vi "Autonomous Independent.vi"() -> ()   [LabVIEW 2014]
doc: "This VI is called when autonomous begins, and will automatically be terminated when autonomous ends. You can carry out timed or sensor driven robot movement independently without needing to return to the caller."
uses:
  <vilib>/Rock Robotics/WPI/Joystick/WPI_JoystickGetSetRefNum.vi
panel:
  out "Stage 3":dbl
  out "Stage 8":dbl
  out "Stage 7":dbl
  out "Stage 6":dbl
  out "Stage 5":dbl
  out "Stage 4":dbl
  out "Stage 2":dbl
  out "Stage":dbl
  out "Right Distance 4":dbl
  out "Left Distance 4":dbl
  out "Elev Height 6":dbl
  out "Left Distance 6":dbl
  out "Right Distance 2":dbl
  out "Left Distance 2":dbl
  out "Right Distance 8":dbl
  out "Left Distance 8":dbl
  out "Right Distance 5":dbl
  out "Left Distance 5":dbl
  out "Right Distance 2":dbl
  out "Left Distance 2":dbl
  out "Right Distance":dbl
  out "Left Distance":dbl
  in  "Arm Control 3":bool
  in  "Right Side Speed 3":dbl
  in  "Left Side Speed 3":dbl
  in  "Elevator Height 4":dbl
  # "Be sure to right-click and choose Data Operations>>Make Current Value default if you want to save the array values with the VI"
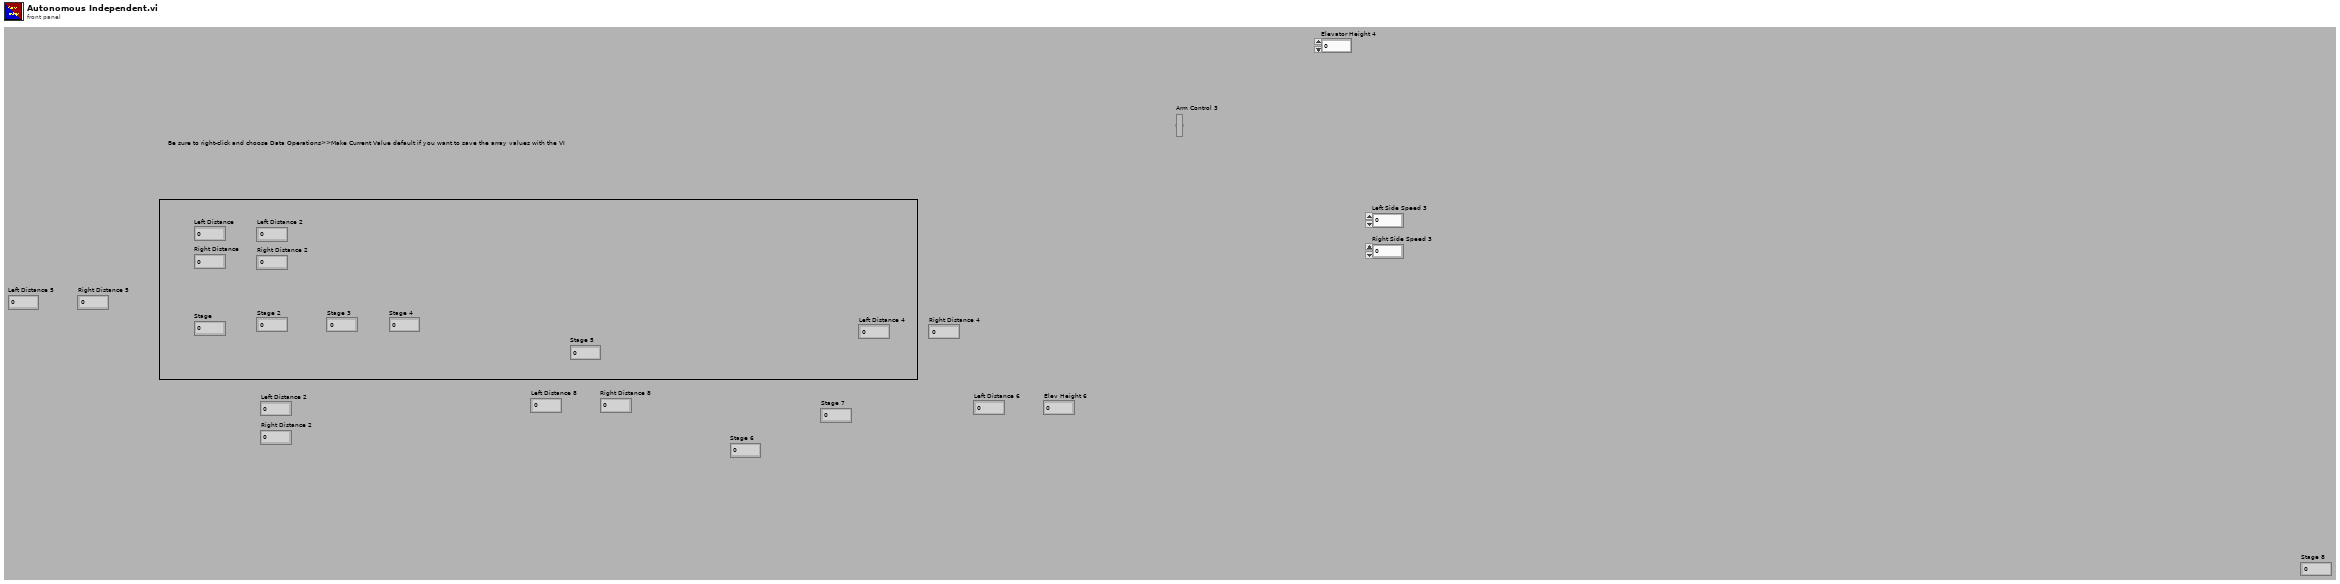
[diagram p1: front panel]
types:
  T1 = cluster{"Encoder Alarm Status":string, "Encoder Distance":dbl, "Encoder Direction":string, "Encoder Rate (distance/sec)":dbl}
  T2 = typedef "WPI_JoystickDevRef.ctl" = cluster{"Device":T3}
  T3 = typedef "WPI_JoystickDeviceEnum.ctl" = enum16{"USB 0", "USB 1", "USB 2", "USB 3", "USB 4", "USB 5"}
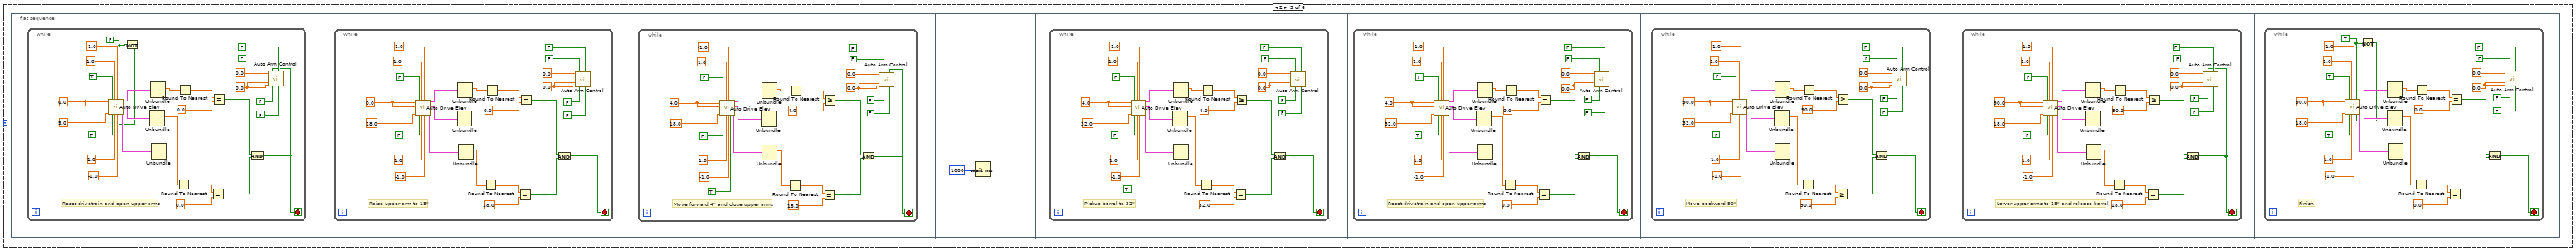
[diagram p3: hidden frame]
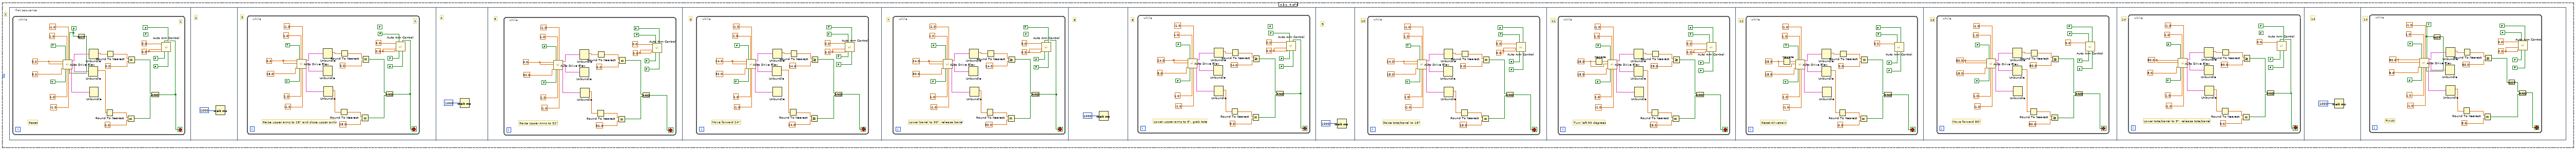
[diagram p4: hidden frame]
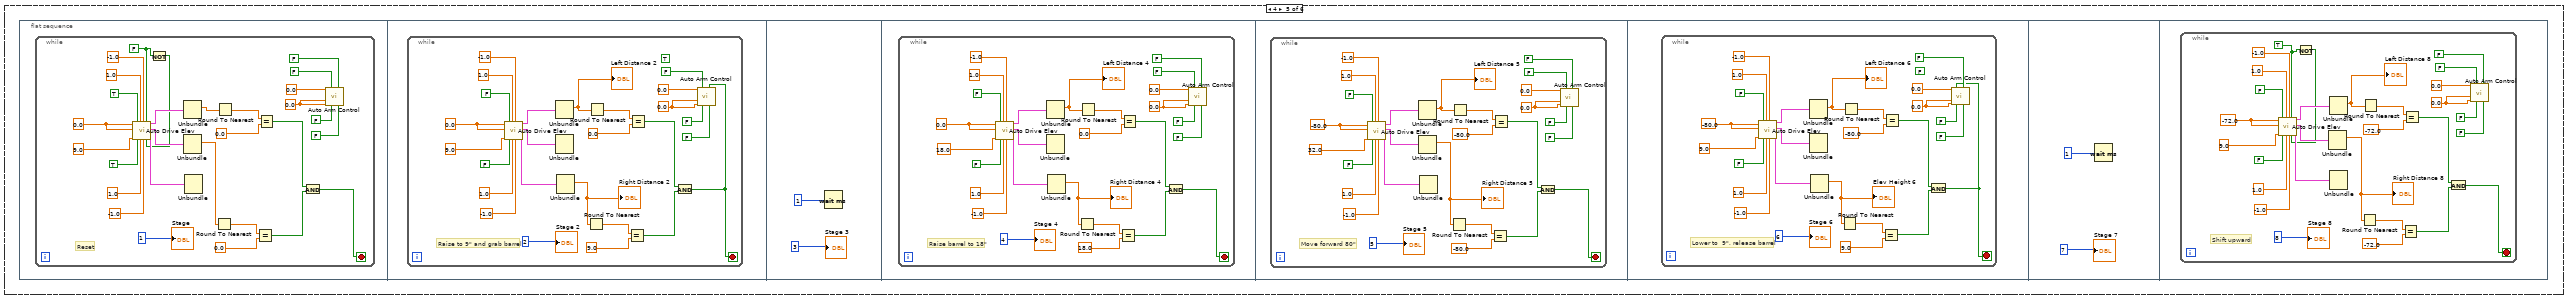
[diagram p5: hidden frame]
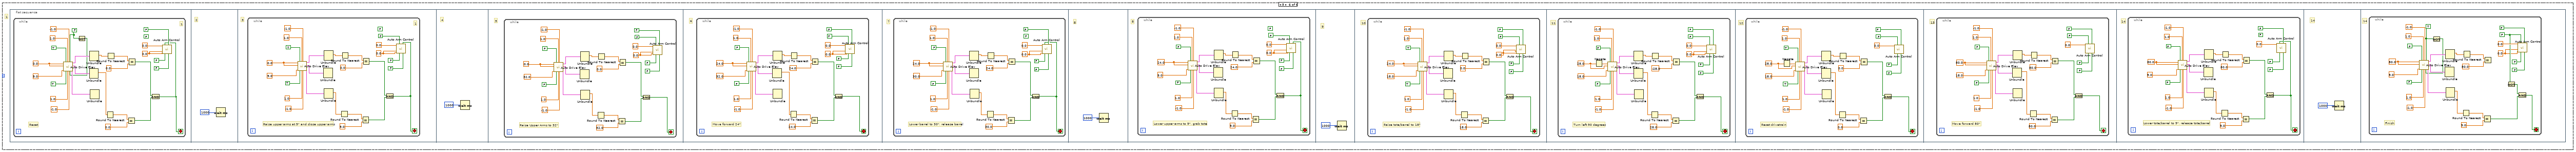
[diagram p6: hidden frame]
diagram:
  (unwired) "This function is run in parallel when the autonomous period begins. It will be terminated automatically when the period ends.\n\nNote that all Driver Station inputs are automatically latched and will not change once auto begins."
  # "Auto Modes\n\n0: Do Nothing\n1: Robot to AutoZone\n2: Barrel to AutoZone\n3: Barrel/Tote to AutoZone\n4: Barrel to AutoZone 2\n5: Discovery World"
  # "Every 20ms, report that we are running autonomous\ncode. Loop will abort the same time as the VI."
  # "This gives you the joystick value\nthat is often the throttle"
  # "This tells you the driver position\nand alliance color"
  n1 = case shown="1" 1 {
    frame 0, Default {
    }
    frame 1 {
      n2 = flat-sequence {
        frame #0 {
          n3 = while {
            stop <- w7 stop-if-true
            w11 = FALSE
            w14 = 0.0
            (unwired) FALSE
            w26 = 0.0
            # "Reset"
            n4 = Not(x=w11) -> (.not. x?=w10:bool)
            n5 = call "Auto Drive Elev.vi"("Left Side Speed"=w26, "Right Side Speed"=w26, "Elevator Height"=9.0, "Left Side Reset"=TRUE, "Right Side Reset"=TRUE, "Left Upper Limit"=1.0, "Right Upper Limit"=1.0, "Left Lower Limit"=-1.0, "Right Lower Limit"=-1.0, "Up Shift"=w11, "Down Shift"=w10) -> ("Encoder Status"=w24:T1, "Encoder Status 2"=w23:T1, "Encoder Status 3"=w22:T1)  [unwired: 6 in]
            n6 = Unbundle(w23) -> ("Encoder Distance"=w8:dbl)  [unwired: 3 out]
            "Right Distance" <- w8
            n7 = Unbundle(w24) -> ("Encoder Distance"=w9:dbl)  [unwired: 3 out]
            "Left Distance" <- w9
            n8 = Unbundle(w22) -> ()  [unwired: 4 out]
            n9 = Round To Nearest(number=w8) -> (nearest integer value=w20:dbl)
            n10 = Round To Nearest(number=w9) -> (nearest integer value=w17:dbl)
            n11 = Equal?(x=w20, y=0.0) -> (x = y?=w19:bool)
            n12 = Equal?(x=w17, y=0.0) -> (x = y?=w16:bool)
            n13 = And(x=w16, y=w19) -> (x .and. y?=w7:bool)
            n14 = call "Auto Arm Control.vi"("Upper Arm Rollers"=0.0, "Upper Arms Open"=FALSE, "Upper Arms Close"=w7, "Lower Roller Left"=w14, "Lower Roller Right"=w14, "Lower Arm Extend"=FALSE, "Lower Arm Retract"=FALSE) -> ()  [unwired: 9 in]
          }
        }
        frame #1 {
          n15 = while {
            stop <- w45 stop-if-true
            w37 = 0.0
            w52 = 60.0
            # "Move forward 5'"
            n16 = call "Auto Drive Elev.vi"("Left Side Speed"=w52, "Right Side Speed"=w52, "Elevator Height"=9.0, "Left Side Reset"=FALSE, "Right Side Reset"=FALSE, "Left Upper Limit"=0.3, "Right Upper Limit"=0.3, "Left Lower Limit"=-0.3, "Right Lower Limit"=-0.3) -> ("Encoder Status"=w50:T1, "Encoder Status 2"=w49:T1, "Encoder Status 3"=w48:T1)  [unwired: 8 in]
            n17 = Unbundle(w49) -> ("Encoder Distance"=w34:dbl)  [unwired: 3 out]
            n18 = Unbundle(w50) -> ("Encoder Distance"=w33:dbl)  [unwired: 3 out]
            n19 = Unbundle(w48) -> ()  [unwired: 4 out]
            n20 = Round To Nearest(number=w34) -> (nearest integer value=w46:dbl)
            n21 = Round To Nearest(number=w33) -> (nearest integer value=w42:dbl)
            n22 = Greater Or Equal?(x=w46, y=60.0) -> (x >= y?=w44:bool)
            n23 = Greater Or Equal?(x=w42, y=60.0) -> (x >= y?=w41:bool)
            n24 = And(x=w41, y=w44) -> (x .and. y?=w45:bool)
            n25 = call "Auto Arm Control.vi"("Upper Arm Rollers"=0.0, "Upper Arms Open"=FALSE, "Upper Arms Close"=FALSE, "Lower Roller Left"=w37, "Lower Roller Right"=w37, "Lower Arm Extend"=FALSE, "Lower Arm Retract"=FALSE) -> ()  [unwired: 9 in]
          }
        }
        frame #2 {
          n26 = while {
            stop <- w73 stop-if-true
            w60 = TRUE
            w65 = 0.0
            w80 = 60.0
            # "Shift upward"
            n27 = Not(x=w60) -> (.not. x?=w59:bool)
            n28 = call "Auto Drive Elev.vi"("Left Side Speed"=w80, "Right Side Speed"=w80, "Elevator Height"=9.0, "Left Side Reset"=FALSE, "Right Side Reset"=FALSE, "Left Upper Limit"=0.0, "Right Upper Limit"=0.0, "Left Lower Limit"=0.0, "Right Lower Limit"=0.0, "Up Shift"=w60, "Down Shift"=w59) -> ("Encoder Status"=w78:T1, "Encoder Status 2"=w77:T1, "Encoder Status 3"=w76:T1)  [unwired: 6 in]
            n29 = Unbundle(w77) -> ("Encoder Distance"=w62:dbl)  [unwired: 3 out]
            "Right Distance 2" <- w62
            n30 = Unbundle(w78) -> ("Encoder Distance"=w61:dbl)  [unwired: 3 out]
            "Left Distance 2" <- w61
            n31 = Unbundle(w76) -> ()  [unwired: 4 out]
            n32 = Round To Nearest(number=w62) -> (nearest integer value=w74:dbl)
            n33 = Round To Nearest(number=w61) -> (nearest integer value=w70:dbl)
            n34 = Greater Or Equal?(x=w74, y=60.0) -> (x >= y?=w72:bool)
            n35 = Greater Or Equal?(x=w70, y=60.0) -> (x >= y?=w69:bool)
            n36 = And(x=w69, y=w72) -> (x .and. y?=w73:bool)
            n37 = call "Auto Arm Control.vi"("Upper Arm Rollers"=0.0, "Upper Arms Open"=FALSE, "Upper Arms Close"=FALSE, "Lower Roller Left"=w65, "Lower Roller Right"=w65, "Lower Arm Extend"=FALSE, "Lower Arm Retract"=FALSE) -> ()  [unwired: 9 in]
          }
        }
      }
    }
    frame 2 {
      n38 = flat-sequence {
        frame #0 {
          n39 = while {
            stop <- w92 stop-if-true
            w88 = FALSE
            w89 = 0.0
            (unwired) FALSE
            w107 = 0.0
            # "Reset drivetrain and open upper arms"
            n40 = Not(x=w88) -> (.not. x?=w87:bool)
            n41 = call "Auto Drive Elev.vi"("Left Side Speed"=w107, "Right Side Speed"=w107, "Elevator Height"=9.0, "Left Side Reset"=TRUE, "Right Side Reset"=TRUE, "Left Upper Limit"=1.0, "Right Upper Limit"=1.0, "Left Lower Limit"=-1.0, "Right Lower Limit"=-1.0, "Up Shift"=w88, "Down Shift"=w87) -> ("Encoder Status"=w105:T1, "Encoder Status 2"=w104:T1, "Encoder Status 3"=w103:T1)  [unwired: 6 in]
            n42 = Unbundle(w104) -> ("Encoder Distance"=w100:dbl)  [unwired: 3 out]
            n43 = Unbundle(w105) -> ("Encoder Distance"=w96:dbl)  [unwired: 3 out]
            n44 = Unbundle(w103) -> ()  [unwired: 4 out]
            n45 = Round To Nearest(number=w100) -> (nearest integer value=w101:dbl)
            n46 = Round To Nearest(number=w96) -> (nearest integer value=w97:dbl)
            n47 = Equal?(x=w101, y=0.0) -> (x = y?=w99:bool)
            n48 = Equal?(x=w97, y=0.0) -> (x = y?=w95:bool)
            n49 = And(x=w95, y=w99) -> (x .and. y?=w92:bool)
            n50 = call "Auto Arm Control.vi"("Upper Arm Rollers"=0.0, "Upper Arms Open"=w92, "Upper Arms Close"=FALSE, "Lower Roller Left"=w89, "Lower Roller Right"=w89, "Lower Arm Extend"=FALSE, "Lower Arm Retract"=FALSE) -> ()  [unwired: 9 in]
          }
        }
        frame #1 {
          n51 = while {
            stop <- w126 stop-if-true
            w114 = 0.0
            w133 = 0.0
            # "Raise upper arm to 18\""
            n52 = call "Auto Drive Elev.vi"("Left Side Speed"=w133, "Right Side Speed"=w133, "Elevator Height"=18.0, "Left Side Reset"=FALSE, "Right Side Reset"=FALSE, "Left Upper Limit"=1.0, "Right Upper Limit"=1.0, "Left Lower Limit"=-1.0, "Right Lower Limit"=-1.0) -> ("Encoder Status"=w131:T1, "Encoder Status 2"=w130:T1, "Encoder Status 3"=w129:T1)  [unwired: 8 in]
            n53 = Unbundle(w130) -> ()  [unwired: 4 out]
            n54 = Unbundle(w131) -> ("Encoder Distance"=w122:dbl)  [unwired: 3 out]
            n55 = Unbundle(w129) -> ("Encoder Distance"=w117:dbl)  [unwired: 3 out]
            n56 = Round To Nearest(number=w117) -> (nearest integer value=w127:dbl)
            n57 = Round To Nearest(number=w122) -> (nearest integer value=w123:dbl)
            n58 = Equal?(x=w127, y=18.0) -> (x = y?=w125:bool)
            n59 = Equal?(x=w123, y=0.0) -> (x = y?=w121:bool)
            n60 = And(x=w121, y=w125) -> (x .and. y?=w126:bool)
            n61 = call "Auto Arm Control.vi"("Upper Arm Rollers"=0.0, "Upper Arms Open"=FALSE, "Upper Arms Close"=FALSE, "Lower Roller Left"=w114, "Lower Roller Right"=w114, "Lower Arm Extend"=FALSE, "Lower Arm Retract"=FALSE) -> ()  [unwired: 9 in]
          }
        }
        frame #2 {
          n62 = while {
            stop <- w144 stop-if-true
            w143 = 0.0
            (unwired) FALSE
            w159 = 4.0
            # "Move forward 4\" and close upper arms"
            n63 = call "Auto Drive Elev.vi"("Left Side Speed"=w159, "Right Side Speed"=w159, "Elevator Height"=18.0, "Left Side Reset"=FALSE, "Right Side Reset"=FALSE, "Left Upper Limit"=1.0, "Right Upper Limit"=1.0, "Left Lower Limit"=-1.0, "Right Lower Limit"=-1.0, "Down Shift"=TRUE) -> ("Encoder Status"=w157:T1, "Encoder Status 2"=w156:T1, "Encoder Status 3"=w155:T1)  [unwired: 7 in]
            n64 = Unbundle(w156) -> ()  [unwired: 4 out]
            n65 = Unbundle(w157) -> ("Encoder Distance"=w149:dbl)  [unwired: 3 out]
            n66 = Unbundle(w155) -> ("Encoder Distance"=w145:dbl)  [unwired: 3 out]
            n67 = Round To Nearest(number=w145) -> (nearest integer value=w153:dbl)
            n68 = Round To Nearest(number=w149) -> (nearest integer value=w150:dbl)
            n69 = Equal?(x=w153, y=18.0) -> (x = y?=w152:bool)
            n70 = Greater Or Equal?(x=w150, y=4.0) -> (x >= y?=w148:bool)
            n71 = And(x=w148, y=w152) -> (x .and. y?=w144:bool)
            n72 = call "Auto Arm Control.vi"("Upper Arm Rollers"=0.0, "Upper Arms Open"=FALSE, "Upper Arms Close"=w144, "Lower Roller Left"=w143, "Lower Roller Right"=w143, "Lower Arm Extend"=FALSE, "Lower Arm Retract"=FALSE) -> ()  [unwired: 9 in]
          }
        }
        frame #3 {
          n73 = Wait (ms)(milliseconds to wait=1000) -> ()  [unwired: 1 out]
        }
        frame #4 {
          n74 = while {
            stop <- w173 stop-if-true
            w170 = 0.0
            w187 = 4.0
            # "Pickup barrel to 32\""
            n75 = call "Auto Drive Elev.vi"("Left Side Speed"=w187, "Right Side Speed"=w187, "Elevator Height"=32.0, "Left Side Reset"=FALSE, "Right Side Reset"=FALSE, "Left Upper Limit"=1.0, "Right Upper Limit"=1.0, "Left Lower Limit"=-1.0, "Right Lower Limit"=-1.0, "Down Shift"=TRUE) -> ("Encoder Status"=w185:T1, "Encoder Status 2"=w184:T1, "Encoder Status 3"=w183:T1)  [unwired: 7 in]
            n76 = Unbundle(w184) -> ("Encoder Distance"=w172:dbl)  [unwired: 3 out]
            n77 = Unbundle(w185) -> ("Encoder Distance"=w177:dbl)  [unwired: 3 out]
            n78 = Unbundle(w183) -> ()  [unwired: 4 out]
            n79 = Round To Nearest(number=w172) -> (nearest integer value=w181:dbl)
            n80 = Round To Nearest(number=w177) -> (nearest integer value=w178:dbl)
            n81 = Equal?(x=w181, y=32.0) -> (x = y?=w180:bool)
            n82 = Greater Or Equal?(x=w178, y=4.0) -> (x >= y?=w176:bool)
            n83 = And(x=w176, y=w180) -> (x .and. y?=w173:bool)
            n84 = call "Auto Arm Control.vi"("Upper Arm Rollers"=0.0, "Upper Arms Open"=FALSE, "Upper Arms Close"=FALSE, "Lower Roller Left"=w170, "Lower Roller Right"=w170, "Lower Arm Extend"=FALSE, "Lower Arm Retract"=FALSE) -> ()  [unwired: 9 in]
          }
        }
        frame #5 {
          n85 = while {
            stop <- w198 stop-if-true
            w194 = 0.0
            w213 = 4.0
            # "Reset drivetrain and open upper arms"
            n86 = call "Auto Drive Elev.vi"("Left Side Speed"=w213, "Right Side Speed"=w213, "Elevator Height"=32.0, "Left Side Reset"=TRUE, "Right Side Reset"=TRUE, "Left Upper Limit"=1.0, "Right Upper Limit"=1.0, "Left Lower Limit"=-1.0, "Right Lower Limit"=-1.0) -> ("Encoder Status"=w211:T1, "Encoder Status 2"=w210:T1, "Encoder Status 3"=w209:T1)  [unwired: 8 in]
            n87 = Unbundle(w210) -> ("Encoder Distance"=w206:dbl)  [unwired: 3 out]
            n88 = Unbundle(w211) -> ("Encoder Distance"=w202:dbl)  [unwired: 3 out]
            n89 = Unbundle(w209) -> ()  [unwired: 4 out]
            n90 = Round To Nearest(number=w206) -> (nearest integer value=w207:dbl)
            n91 = Round To Nearest(number=w202) -> (nearest integer value=w203:dbl)
            n92 = Equal?(x=w207, y=0.0) -> (x = y?=w205:bool)
            n93 = Equal?(x=w203, y=0.0) -> (x = y?=w201:bool)
            n94 = And(x=w201, y=w205) -> (x .and. y?=w198:bool)
            n95 = call "Auto Arm Control.vi"("Upper Arm Rollers"=0.0, "Upper Arms Open"=FALSE, "Upper Arms Close"=FALSE, "Lower Roller Left"=w194, "Lower Roller Right"=w194, "Lower Arm Extend"=FALSE, "Lower Arm Retract"=FALSE) -> ()  [unwired: 9 in]
          }
        }
        frame #6 {
          n96 = while {
            stop <- w225 stop-if-true
            w222 = 0.0
            w239 = 90.0
            # "Move backward 90\""
            n97 = call "Auto Drive Elev.vi"("Left Side Speed"=w239, "Right Side Speed"=w239, "Elevator Height"=32.0, "Left Side Reset"=FALSE, "Right Side Reset"=FALSE, "Left Upper Limit"=1.0, "Right Upper Limit"=1.0, "Left Lower Limit"=-1.0, "Right Lower Limit"=-1.0) -> ("Encoder Status"=w237:T1, "Encoder Status 2"=w236:T1, "Encoder Status 3"=w235:T1)  [unwired: 8 in]
            n98 = Unbundle(w236) -> ("Encoder Distance"=w223:dbl)  [unwired: 3 out]
            n99 = Unbundle(w237) -> ("Encoder Distance"=w229:dbl)  [unwired: 3 out]
            n100 = Unbundle(w235) -> ()  [unwired: 4 out]
            n101 = Round To Nearest(number=w223) -> (nearest integer value=w233:dbl)
            n102 = Round To Nearest(number=w229) -> (nearest integer value=w230:dbl)
            n103 = Greater Or Equal?(x=w233, y=90.0) -> (x >= y?=w232:bool)
            n104 = Greater Or Equal?(x=w230, y=90.0) -> (x >= y?=w228:bool)
            n105 = And(x=w228, y=w232) -> (x .and. y?=w225:bool)
            n106 = call "Auto Arm Control.vi"("Upper Arm Rollers"=0.0, "Upper Arms Open"=FALSE, "Upper Arms Close"=FALSE, "Lower Roller Left"=w222, "Lower Roller Right"=w222, "Lower Arm Extend"=FALSE, "Lower Arm Retract"=FALSE) -> ()  [unwired: 9 in]
          }
        }
        frame #7 {
          n107 = while {
            stop <- w249 stop-if-true
            w246 = 0.0
            (unwired) FALSE
            w264 = 90.0
            # "Lower upper arms to 18\" and release barrel"
            n108 = call "Auto Drive Elev.vi"("Left Side Speed"=w264, "Right Side Speed"=w264, "Elevator Height"=18.0, "Left Side Reset"=FALSE, "Right Side Reset"=FALSE, "Left Upper Limit"=1.0, "Right Upper Limit"=1.0, "Left Lower Limit"=-1.0, "Right Lower Limit"=-1.0) -> ("Encoder Status"=w262:T1, "Encoder Status 2"=w261:T1, "Encoder Status 3"=w260:T1)  [unwired: 8 in]
            n109 = Unbundle(w261) -> ()  [unwired: 4 out]
            n110 = Unbundle(w262) -> ("Encoder Distance"=w254:dbl)  [unwired: 3 out]
            n111 = Unbundle(w260) -> ("Encoder Distance"=w250:dbl)  [unwired: 3 out]
            n112 = Round To Nearest(number=w250) -> (nearest integer value=w258:dbl)
            n113 = Round To Nearest(number=w254) -> (nearest integer value=w255:dbl)
            n114 = Equal?(x=w258, y=18.0) -> (x = y?=w257:bool)
            n115 = Greater Or Equal?(x=w255, y=90.0) -> (x >= y?=w253:bool)
            n116 = And(x=w253, y=w257) -> (x .and. y?=w249:bool)
            n117 = call "Auto Arm Control.vi"("Upper Arm Rollers"=0.0, "Upper Arms Open"=w249, "Upper Arms Close"=FALSE, "Lower Roller Left"=w246, "Lower Roller Right"=w246, "Lower Arm Extend"=FALSE, "Lower Arm Retract"=FALSE) -> ()  [unwired: 9 in]
          }
        }
        frame #8 {
          n118 = while {
            stop <- w278 stop-if-true
            w271 = TRUE
            w273 = 0.0
            w292 = 90.0
            # "Finish"
            n119 = Not(x=w271) -> (.not. x?=w272:bool)
            n120 = call "Auto Drive Elev.vi"("Left Side Speed"=w292, "Right Side Speed"=w292, "Elevator Height"=18.0, "Left Side Reset"=TRUE, "Right Side Reset"=TRUE, "Left Upper Limit"=1.0, "Right Upper Limit"=1.0, "Left Lower Limit"=-1.0, "Right Lower Limit"=-1.0, "Up Shift"=w271, "Down Shift"=w272) -> ("Encoder Status"=w290:T1, "Encoder Status 2"=w289:T1, "Encoder Status 3"=w288:T1)  [unwired: 6 in]
            n121 = Unbundle(w289) -> ("Encoder Distance"=w277:dbl)  [unwired: 3 out]
            n122 = Unbundle(w290) -> ("Encoder Distance"=w282:dbl)  [unwired: 3 out]
            n123 = Unbundle(w288) -> ()  [unwired: 4 out]
            n124 = Round To Nearest(number=w277) -> (nearest integer value=w286:dbl)
            n125 = Round To Nearest(number=w282) -> (nearest integer value=w283:dbl)
            n126 = Equal?(x=w286, y=0.0) -> (x = y?=w285:bool)
            n127 = Equal?(x=w283, y=0.0) -> (x = y?=w281:bool)
            n128 = And(x=w281, y=w285) -> (x .and. y?=w278:bool)
            n129 = call "Auto Arm Control.vi"("Upper Arm Rollers"=0.0, "Upper Arms Open"=FALSE, "Upper Arms Close"=FALSE, "Lower Roller Left"=w273, "Lower Roller Right"=w273, "Lower Arm Extend"=FALSE, "Lower Arm Retract"=FALSE) -> ()  [unwired: 9 in]
          }
        }
      }
    }
    frame 3 {
      # "1"
      n130 = flat-sequence {
        frame #0 {
          # "1"
          n131 = while {
            stop <- w301 stop-if-true
            w299 = FALSE
            w303 = 0.0
            (unwired) FALSE
            w319 = 0.0
            # "Reset"
            n132 = Not(x=w299) -> (.not. x?=w300:bool)
            n133 = call "Auto Drive Elev.vi"("Left Side Speed"=w319, "Right Side Speed"=w319, "Elevator Height"=9.0, "Left Side Reset"=TRUE, "Right Side Reset"=TRUE, "Left Upper Limit"=1.0, "Right Upper Limit"=1.0, "Left Lower Limit"=-1.0, "Right Lower Limit"=-1.0, "Up Shift"=w299, "Down Shift"=w300) -> ("Encoder Status"=w317:T1, "Encoder Status 2"=w316:T1, "Encoder Status 3"=w315:T1)  [unwired: 6 in]
            n134 = Unbundle(w316) -> ("Encoder Distance"=w312:dbl)  [unwired: 3 out]
            n135 = Unbundle(w317) -> ("Encoder Distance"=w308:dbl)  [unwired: 3 out]
            n136 = Unbundle(w315) -> ()  [unwired: 4 out]
            n137 = Round To Nearest(number=w312) -> (nearest integer value=w313:dbl)
            n138 = Round To Nearest(number=w308) -> (nearest integer value=w309:dbl)
            n139 = Equal?(x=w313, y=0.0) -> (x = y?=w311:bool)
            n140 = Equal?(x=w309, y=0.0) -> (x = y?=w307:bool)
            n141 = And(x=w307, y=w311) -> (x .and. y?=w301:bool)
            n142 = call "Auto Arm Control.vi"("Upper Arm Rollers"=0.0, "Upper Arms Open"=w301, "Upper Arms Close"=FALSE, "Lower Roller Left"=w303, "Lower Roller Right"=w303, "Lower Arm Extend"=FALSE, "Lower Arm Retract"=FALSE) -> ()  [unwired: 9 in]
          }
        }
        frame #1 {
          # "2"
          n143 = Wait (ms)(milliseconds to wait=1000) -> ()  [unwired: 1 out]
        }
        frame #2 {
          # "3"
          # "1"
          n144 = while {
            stop <- w328 stop-if-true
            w329 = 0.0
            (unwired) FALSE
            w345 = 0.0
            # "Raise upper arms to 18\" and close upper arms"
            n145 = call "Auto Drive Elev.vi"("Left Side Speed"=w345, "Right Side Speed"=w345, "Elevator Height"=18.0, "Left Side Reset"=TRUE, "Right Side Reset"=TRUE, "Left Upper Limit"=1.0, "Right Upper Limit"=1.0, "Left Lower Limit"=-1.0, "Right Lower Limit"=-1.0) -> ("Encoder Status"=w343:T1, "Encoder Status 2"=w342:T1, "Encoder Status 3"=w341:T1)  [unwired: 8 in]
            n146 = Unbundle(w342) -> ()  [unwired: 4 out]
            n147 = Unbundle(w343) -> ("Encoder Distance"=w335:dbl)  [unwired: 3 out]
            n148 = Unbundle(w341) -> ("Encoder Distance"=w332:dbl)  [unwired: 3 out]
            n149 = Round To Nearest(number=w332) -> (nearest integer value=w339:dbl)
            n150 = Round To Nearest(number=w335) -> (nearest integer value=w336:dbl)
            n151 = Equal?(x=w339, y=18.0) -> (x = y?=w338:bool)
            n152 = Equal?(x=w336, y=0.0) -> (x = y?=w327:bool)
            n153 = And(x=w327, y=w338) -> (x .and. y?=w328:bool)
            n154 = call "Auto Arm Control.vi"("Upper Arm Rollers"=0.0, "Upper Arms Open"=FALSE, "Upper Arms Close"=w328, "Lower Roller Left"=w329, "Lower Roller Right"=w329, "Lower Arm Extend"=FALSE, "Lower Arm Retract"=FALSE) -> ()  [unwired: 9 in]
          }
        }
        frame #3 {
          # "4"
          n155 = Wait (ms)(milliseconds to wait=1000) -> ()  [unwired: 1 out]
        }
        frame #4 {
          # "5"
          n156 = while {
            stop <- w365 stop-if-true
            w354 = 0.0
            w372 = 0.0
            # "Raise Upper Arms to 32\""
            n157 = call "Auto Drive Elev.vi"("Left Side Speed"=w372, "Right Side Speed"=w372, "Elevator Height"=32.0, "Left Side Reset"=FALSE, "Right Side Reset"=FALSE, "Left Upper Limit"=1.0, "Right Upper Limit"=1.0, "Left Lower Limit"=-1.0, "Right Lower Limit"=-1.0) -> ("Encoder Status"=w370:T1, "Encoder Status 2"=w369:T1, "Encoder Status 3"=w368:T1)  [unwired: 8 in]
            n158 = Unbundle(w369) -> ()  [unwired: 4 out]
            n159 = Unbundle(w370) -> ("Encoder Distance"=w361:dbl)  [unwired: 3 out]
            n160 = Unbundle(w368) -> ("Encoder Distance"=w356:dbl)  [unwired: 3 out]
            n161 = Round To Nearest(number=w356) -> (nearest integer value=w366:dbl)
            n162 = Round To Nearest(number=w361) -> (nearest integer value=w362:dbl)
            n163 = Equal?(x=w366, y=32.0) -> (x = y?=w364:bool)
            n164 = Equal?(x=w362, y=0.0) -> (x = y?=w360:bool)
            n165 = And(x=w360, y=w364) -> (x .and. y?=w365:bool)
            n166 = call "Auto Arm Control.vi"("Upper Arm Rollers"=0.0, "Upper Arms Open"=FALSE, "Upper Arms Close"=FALSE, "Lower Roller Left"=w354, "Lower Roller Right"=w354, "Lower Arm Extend"=FALSE, "Lower Arm Retract"=FALSE) -> ()  [unwired: 9 in]
          }
        }
        frame #5 {
          # "6"
          n167 = while {
            stop <- w390 stop-if-true
            w379 = 0.0
            w398 = 24.0
            # "Move forward 24\""
            n168 = call "Auto Drive Elev.vi"("Left Side Speed"=w398, "Right Side Speed"=w398, "Elevator Height"=32.0, "Left Side Reset"=FALSE, "Right Side Reset"=FALSE, "Left Upper Limit"=1.0, "Right Upper Limit"=1.0, "Left Lower Limit"=-1.0, "Right Lower Limit"=-1.0) -> ("Encoder Status"=w396:T1, "Encoder Status 2"=w395:T1, "Encoder Status 3"=w394:T1)  [unwired: 8 in]
            n169 = Unbundle(w395) -> ("Encoder Distance"=w391:dbl)  [unwired: 3 out]
            n170 = Unbundle(w396) -> ("Encoder Distance"=w386:dbl)  [unwired: 3 out]
            n171 = Unbundle(w394) -> ()  [unwired: 4 out]
            n172 = Round To Nearest(number=w391) -> (nearest integer value=w392:dbl)
            n173 = Round To Nearest(number=w386) -> (nearest integer value=w387:dbl)
            n174 = Greater Or Equal?(x=w392, y=24.0) -> (x >= y?=w389:bool)
            n175 = Greater Or Equal?(x=w387, y=24.0) -> (x >= y?=w385:bool)
            n176 = And(x=w385, y=w389) -> (x .and. y?=w390:bool)
            n177 = call "Auto Arm Control.vi"("Upper Arm Rollers"=0.0, "Upper Arms Open"=FALSE, "Upper Arms Close"=FALSE, "Lower Roller Left"=w379, "Lower Roller Right"=w379, "Lower Arm Extend"=FALSE, "Lower Arm Retract"=FALSE) -> ()  [unwired: 9 in]
          }
        }
        frame #6 {
          # "7"
          n178 = while {
            stop <- w405 stop-if-true
            w406 = 0.0
            (unwired) FALSE
            w423 = 24.0
            # "Lower barrel to 30\", release barrel"
            n179 = call "Auto Drive Elev.vi"("Left Side Speed"=w423, "Right Side Speed"=w423, "Elevator Height"=30.0, "Left Side Reset"=FALSE, "Right Side Reset"=FALSE, "Left Upper Limit"=1.0, "Right Upper Limit"=1.0, "Left Lower Limit"=-1.0, "Right Lower Limit"=-1.0) -> ("Encoder Status"=w421:T1, "Encoder Status 2"=w420:T1, "Encoder Status 3"=w419:T1)  [unwired: 8 in]
            n180 = Unbundle(w420) -> ()  [unwired: 4 out]
            n181 = Unbundle(w421) -> ("Encoder Distance"=w413:dbl)  [unwired: 3 out]
            n182 = Unbundle(w419) -> ("Encoder Distance"=w409:dbl)  [unwired: 3 out]
            n183 = Round To Nearest(number=w409) -> (nearest integer value=w417:dbl)
            n184 = Round To Nearest(number=w413) -> (nearest integer value=w414:dbl)
            n185 = Equal?(x=w417, y=30.0) -> (x = y?=w416:bool)
            n186 = Greater Or Equal?(x=w414, y=24.0) -> (x >= y?=w412:bool)
            n187 = And(x=w412, y=w416) -> (x .and. y?=w405:bool)
            n188 = call "Auto Arm Control.vi"("Upper Arm Rollers"=0.0, "Upper Arms Open"=w405, "Upper Arms Close"=FALSE, "Lower Roller Left"=w406, "Lower Roller Right"=w406, "Lower Arm Extend"=FALSE, "Lower Arm Retract"=FALSE) -> ()  [unwired: 9 in]
          }
        }
        frame #7 {
          # "8"
          n189 = Wait (ms)(milliseconds to wait=1000) -> ()  [unwired: 1 out]
        }
        frame #8 {
          # "8"
          n190 = while {
            stop <- w431 stop-if-true
            w434 = 0.0
            (unwired) FALSE
            w449 = 24.0
            # "Lower upper arms to 9\", grab tote"
            n191 = call "Auto Drive Elev.vi"("Left Side Speed"=w449, "Right Side Speed"=w449, "Elevator Height"=9.0, "Left Side Reset"=FALSE, "Right Side Reset"=FALSE, "Left Upper Limit"=1.0, "Right Upper Limit"=1.0, "Left Lower Limit"=-1.0, "Right Lower Limit"=-1.0) -> ("Encoder Status"=w447:T1, "Encoder Status 2"=w446:T1, "Encoder Status 3"=w445:T1)  [unwired: 8 in]
            n192 = Unbundle(w446) -> ()  [unwired: 4 out]
            n193 = Unbundle(w447) -> ("Encoder Distance"=w439:dbl)  [unwired: 3 out]
            n194 = Unbundle(w445) -> ("Encoder Distance"=w435:dbl)  [unwired: 3 out]
            n195 = Round To Nearest(number=w435) -> (nearest integer value=w443:dbl)
            n196 = Round To Nearest(number=w439) -> (nearest integer value=w440:dbl)
            n197 = Equal?(x=w443, y=9.0) -> (x = y?=w442:bool)
            n198 = Greater Or Equal?(x=w440, y=24.0) -> (x >= y?=w438:bool)
            n199 = And(x=w438, y=w442) -> (x .and. y?=w431:bool)
            n200 = call "Auto Arm Control.vi"("Upper Arm Rollers"=0.0, "Upper Arms Open"=FALSE, "Upper Arms Close"=w431, "Lower Roller Left"=w434, "Lower Roller Right"=w434, "Lower Arm Extend"=FALSE, "Lower Arm Retract"=FALSE) -> ()  [unwired: 9 in]
          }
        }
        frame #9 {
          # "9"
          n201 = Wait (ms)(milliseconds to wait=1000) -> ()  [unwired: 1 out]
        }
        frame #10 {
          # "10"
          n202 = while {
            stop <- w469 stop-if-true
            w457 = 0.0
            w476 = 24.0
            # "Raise tote/barrel to 18\""
            n203 = call "Auto Drive Elev.vi"("Left Side Speed"=w476, "Right Side Speed"=w476, "Elevator Height"=18.0, "Left Side Reset"=TRUE, "Right Side Reset"=TRUE, "Left Upper Limit"=1.0, "Right Upper Limit"=1.0, "Left Lower Limit"=-1.0, "Right Lower Limit"=-1.0) -> ("Encoder Status"=w474:T1, "Encoder Status 2"=w473:T1, "Encoder Status 3"=w472:T1)  [unwired: 8 in]
            n204 = Unbundle(w473) -> ()  [unwired: 4 out]
            n205 = Unbundle(w474) -> ("Encoder Distance"=w465:dbl)  [unwired: 3 out]
            n206 = Unbundle(w472) -> ("Encoder Distance"=w460:dbl)  [unwired: 3 out]
            n207 = Round To Nearest(number=w460) -> (nearest integer value=w470:dbl)
            n208 = Round To Nearest(number=w465) -> (nearest integer value=w466:dbl)
            n209 = Equal?(x=w470, y=18.0) -> (x = y?=w468:bool)
            n210 = Equal?(x=w466, y=0.0) -> (x = y?=w461:bool)
            n211 = And(x=w461, y=w468) -> (x .and. y?=w469:bool)
            n212 = call "Auto Arm Control.vi"("Upper Arm Rollers"=0.0, "Upper Arms Open"=FALSE, "Upper Arms Close"=FALSE, "Lower Roller Left"=w457, "Lower Roller Right"=w457, "Lower Arm Extend"=FALSE, "Lower Arm Retract"=FALSE) -> ()  [unwired: 9 in]
          }
        }
        frame #11 {
          # "11"
          n213 = while {
            stop <- w497 stop-if-true
            w483 = 0.0
            w486 = 28.0
            # "Turn left 90 degrees"
            n214 = Negate(x=w486) -> (-x=w487:dbl)
            n215 = call "Auto Drive Elev.vi"("Left Side Speed"=w487, "Right Side Speed"=w486, "Elevator Height"=18.0, "Left Side Reset"=FALSE, "Right Side Reset"=FALSE, "Left Upper Limit"=1.0, "Right Upper Limit"=1.0, "Left Lower Limit"=-1.0, "Right Lower Limit"=-1.0) -> ("Encoder Status"=w502:T1, "Encoder Status 2"=w501:T1, "Encoder Status 3"=w500:T1)  [unwired: 8 in]
            n216 = Unbundle(w501) -> ("Encoder Distance"=w488:dbl)  [unwired: 3 out]
            n217 = Unbundle(w502) -> ("Encoder Distance"=w493:dbl)  [unwired: 3 out]
            n218 = Unbundle(w500) -> ()  [unwired: 4 out]
            n219 = Round To Nearest(number=w488) -> (nearest integer value=w498:dbl)
            n220 = Round To Nearest(number=w493) -> (nearest integer value=w494:dbl)
            n221 = Equal?(x=w498, y=28.0) -> (x = y?=w496:bool)
            n222 = Greater Or Equal?(x=w494, y=28.0) -> (x >= y?=w489:bool)
            n223 = And(x=w489, y=w496) -> (x .and. y?=w497:bool)
            n224 = call "Auto Arm Control.vi"("Upper Arm Rollers"=0.0, "Upper Arms Open"=FALSE, "Upper Arms Close"=FALSE, "Lower Roller Left"=w483, "Lower Roller Right"=w483, "Lower Arm Extend"=FALSE, "Lower Arm Retract"=FALSE) -> ()  [unwired: 9 in]
          }
        }
        frame #12 {
          # "12"
          n225 = while {
            stop <- w523 stop-if-true
            w512 = 28.0
            # "Reset drivetrain"
            n226 = Negate(x=w512) -> (-x=w513:dbl)
            n227 = call "Auto Drive Elev.vi"("Left Side Speed"=w513, "Right Side Speed"=w512, "Elevator Height"=18.0, "Left Side Reset"=TRUE, "Right Side Reset"=TRUE, "Left Upper Limit"=1.0, "Right Upper Limit"=1.0, "Left Lower Limit"=-1.0, "Right Lower Limit"=-1.0) -> ("Encoder Status"=w528:T1, "Encoder Status 2"=w527:T1, "Encoder Status 3"=w526:T1)  [unwired: 8 in]
            n228 = Unbundle(w527) -> ("Encoder Distance"=w514:dbl)  [unwired: 3 out]
            n229 = Unbundle(w528) -> ("Encoder Distance"=w519:dbl)  [unwired: 3 out]
            n230 = Unbundle(w526) -> ()  [unwired: 4 out]
            n231 = Round To Nearest(number=w514) -> (nearest integer value=w524:dbl)
            n232 = Round To Nearest(number=w519) -> (nearest integer value=w520:dbl)
            n233 = Equal?(x=w524, y=0.0) -> (x = y?=w522:bool)
            n234 = Equal?(x=w520, y=0.0) -> (x = y?=w515:bool)
            n235 = And(x=w515, y=w522) -> (x .and. y?=w523:bool)
            n236 = call "Auto Arm Control.vi"("Upper Arm Rollers"=0.0, "Upper Arms Open"=FALSE, "Upper Arms Close"=FALSE, "Lower Arm Extend"=FALSE, "Lower Arm Retract"=FALSE) -> ()  [unwired: 11 in]
          }
        }
        frame #13 {
          # "13"
          n237 = while {
            stop <- w548 stop-if-true
            w538 = 80.0
            # "Move forward 80\""
            n238 = call "Auto Drive Elev.vi"("Left Side Speed"=w538, "Right Side Speed"=w538, "Elevator Height"=18.0, "Left Side Reset"=FALSE, "Right Side Reset"=FALSE, "Left Upper Limit"=1.0, "Right Upper Limit"=1.0, "Left Lower Limit"=-1.0, "Right Lower Limit"=-1.0) -> ("Encoder Status"=w553:T1, "Encoder Status 2"=w552:T1, "Encoder Status 3"=w551:T1)  [unwired: 8 in]
            n239 = Unbundle(w552) -> ("Encoder Distance"=w539:dbl)  [unwired: 3 out]
            n240 = Unbundle(w553) -> ("Encoder Distance"=w544:dbl)  [unwired: 3 out]
            n241 = Unbundle(w551) -> ()  [unwired: 4 out]
            n242 = Round To Nearest(number=w539) -> (nearest integer value=w549:dbl)
            n243 = Round To Nearest(number=w544) -> (nearest integer value=w545:dbl)
            n244 = Greater Or Equal?(x=w549, y=80.0) -> (x >= y?=w547:bool)
            n245 = Greater Or Equal?(x=w545, y=80.0) -> (x >= y?=w540:bool)
            n246 = And(x=w540, y=w547) -> (x .and. y?=w548:bool)
            n247 = call "Auto Arm Control.vi"("Upper Arm Rollers"=0.0, "Upper Arms Open"=FALSE, "Upper Arms Close"=FALSE, "Lower Arm Extend"=FALSE, "Lower Arm Retract"=FALSE) -> ()  [unwired: 11 in]
          }
        }
        frame #14 {
          # "14"
          n248 = while {
            stop <- w561 stop-if-true
            (unwired) FALSE
            w565 = 80.0
            # "Lower tote/barrel to 9\", release tote/barrel"
            n249 = call "Auto Drive Elev.vi"("Left Side Speed"=w565, "Right Side Speed"=w565, "Elevator Height"=9.0, "Left Side Reset"=FALSE, "Right Side Reset"=FALSE, "Left Upper Limit"=1.0, "Right Upper Limit"=1.0, "Left Lower Limit"=-1.0, "Right Lower Limit"=-1.0) -> ("Encoder Status"=w577:T1, "Encoder Status 2"=w576:T1, "Encoder Status 3"=w575:T1)  [unwired: 8 in]
            n250 = Unbundle(w576) -> ()  [unwired: 4 out]
            n251 = Unbundle(w577) -> ("Encoder Distance"=w569:dbl)  [unwired: 3 out]
            n252 = Unbundle(w575) -> ("Encoder Distance"=w564:dbl)  [unwired: 3 out]
            n253 = Round To Nearest(number=w564) -> (nearest integer value=w573:dbl)
            n254 = Round To Nearest(number=w569) -> (nearest integer value=w570:dbl)
            n255 = Equal?(x=w573, y=9.0) -> (x = y?=w572:bool)
            n256 = Greater Or Equal?(x=w570, y=80.0) -> (x >= y?=w566:bool)
            n257 = And(x=w566, y=w572) -> (x .and. y?=w561:bool)
            n258 = call "Auto Arm Control.vi"("Upper Arm Rollers"=0.0, "Upper Arms Open"=w561, "Upper Arms Close"=FALSE, "Lower Arm Extend"=FALSE, "Lower Arm Retract"=FALSE) -> ()  [unwired: 11 in]
          }
        }
        frame #15 {
          # "14"
          n259 = Wait (ms)(milliseconds to wait=1000) -> ()  [unwired: 1 out]
        }
        frame #16 {
          # "14"
          n260 = while {
            stop <- w602 stop-if-true
            w587 = TRUE
            w589 = 0.0
            w595 = 80.0
            # "Finish"
            n261 = Not(x=w587) -> (.not. x?=w588:bool)
            n262 = call "Auto Drive Elev.vi"("Left Side Speed"=w595, "Right Side Speed"=w595, "Elevator Height"=9.0, "Left Side Reset"=FALSE, "Right Side Reset"=FALSE, "Left Upper Limit"=1.0, "Right Upper Limit"=1.0, "Left Lower Limit"=-1.0, "Right Lower Limit"=-1.0, "Up Shift"=w587, "Down Shift"=w588) -> ("Encoder Status"=w607:T1, "Encoder Status 2"=w606:T1, "Encoder Status 3"=w605:T1)  [unwired: 6 in]
            n263 = Unbundle(w606) -> ()  [unwired: 4 out]
            n264 = Unbundle(w607) -> ("Encoder Distance"=w598:dbl)  [unwired: 3 out]
            n265 = Unbundle(w605) -> ("Encoder Distance"=w594:dbl)  [unwired: 3 out]
            n266 = Round To Nearest(number=w594) -> (nearest integer value=w603:dbl)
            n267 = Round To Nearest(number=w598) -> (nearest integer value=w599:dbl)
            n268 = Equal?(x=w603, y=9.0) -> (x = y?=w601:bool)
            n269 = Greater Or Equal?(x=w599, y=80.0) -> (x >= y?=w586:bool)
            n270 = Not(x=w586) -> (.not. x?=w593:bool)
            n271 = And(x=w593, y=w601) -> (x .and. y?=w602:bool)
            n272 = call "Auto Arm Control.vi"("Upper Arm Rollers"=0.0, "Upper Arms Open"=FALSE, "Upper Arms Close"=FALSE, "Lower Roller Left"=w589, "Lower Roller Right"=w589, "Lower Arm Extend"=FALSE, "Lower Arm Retract"=FALSE) -> ()  [unwired: 9 in]
          }
        }
      }
    }
    frame 4 {
      n273 = flat-sequence {
        frame #0 {
          n274 = while {
            stop <- w629 stop-if-true
            w617 = FALSE
            w620 = 0.0
            w637 = 0.0
            # "Reset"
            n275 = Not(x=w617) -> (.not. x?=w616:bool)
            n276 = call "Auto Drive Elev.vi"("Left Side Speed"=w637, "Right Side Speed"=w637, "Elevator Height"=9.0, "Left Side Reset"=TRUE, "Right Side Reset"=TRUE, "Left Upper Limit"=1.0, "Right Upper Limit"=1.0, "Left Lower Limit"=-1.0, "Right Lower Limit"=-1.0, "Up Shift"=w617, "Down Shift"=w616) -> ("Encoder Status"=w635:T1, "Encoder Status 2"=w634:T1, "Encoder Status 3"=w633:T1)  [unwired: 6 in]
            n277 = Unbundle(w634) -> ("Encoder Distance"=w630:dbl)  [unwired: 3 out]
            n278 = Unbundle(w635) -> ("Encoder Distance"=w625:dbl)  [unwired: 3 out]
            n279 = Unbundle(w633) -> ()  [unwired: 4 out]
            n280 = Round To Nearest(number=w630) -> (nearest integer value=w631:dbl)
            n281 = Round To Nearest(number=w625) -> (nearest integer value=w626:dbl)
            n282 = Equal?(x=w631, y=0.0) -> (x = y?=w628:bool)
            n283 = Equal?(x=w626, y=0.0) -> (x = y?=w624:bool)
            n284 = And(x=w624, y=w628) -> (x .and. y?=w629:bool)
            n285 = call "Auto Arm Control.vi"("Upper Arm Rollers"=0.0, "Upper Arms Open"=FALSE, "Upper Arms Close"=FALSE, "Lower Roller Left"=w620, "Lower Roller Right"=w620, "Lower Arm Extend"=FALSE, "Lower Arm Retract"=FALSE) -> ()  [unwired: 9 in]
            "Stage" <- 1
          }
        }
        frame #1 {
          n286 = while {
            stop <- w644 stop-if-true
            w650 = 0.0
            (unwired) TRUE
            w663 = 0.0
            # "Raise to 9\" and grab barrel"
            n287 = call "Auto Drive Elev.vi"("Left Side Speed"=w663, "Right Side Speed"=w663, "Elevator Height"=9.0, "Left Side Reset"=FALSE, "Right Side Reset"=FALSE, "Left Upper Limit"=1.0, "Right Upper Limit"=1.0, "Left Lower Limit"=-1.0, "Right Lower Limit"=-1.0) -> ("Encoder Status"=w661:T1, "Encoder Status 2"=w660:T1, "Encoder Status 3"=w659:T1)  [unwired: 8 in]
            n288 = Unbundle(w660) -> ()  [unwired: 4 out]
            n289 = Unbundle(w661) -> ("Encoder Distance"=w647:dbl)  [unwired: 3 out]
            "Left Distance 2" <- w647
            n290 = Unbundle(w659) -> ("Encoder Distance"=w645:dbl)  [unwired: 3 out]
            "Right Distance 2" <- w645
            n291 = Round To Nearest(number=w645) -> (nearest integer value=w657:dbl)
            n292 = Round To Nearest(number=w647) -> (nearest integer value=w654:dbl)
            n293 = Equal?(x=w657, y=9.0) -> (x = y?=w656:bool)
            n294 = Equal?(x=w654, y=0.0) -> (x = y?=w653:bool)
            n295 = And(x=w653, y=w656) -> (x .and. y?=w644:bool)
            n296 = call "Auto Arm Control.vi"("Upper Arm Rollers"=0.0, "Upper Arms Open"=FALSE, "Upper Arms Close"=w644, "Lower Roller Left"=w650, "Lower Roller Right"=w650, "Lower Arm Extend"=FALSE, "Lower Arm Retract"=FALSE) -> ()  [unwired: 9 in]
            "Stage 2" <- 2
          }
        }
        frame #2 {
          n297 = Wait (ms)(milliseconds to wait=1) -> ()  [unwired: 1 out]
          "Stage 3" <- 3
        }
        frame #3 {
          n298 = while {
            stop <- w675 stop-if-true
            w679 = 0.0
            w692 = 0.0
            # "Raise barrel to 18\""
            n299 = call "Auto Drive Elev.vi"("Left Side Speed"=w692, "Right Side Speed"=w692, "Elevator Height"=18.0, "Left Side Reset"=FALSE, "Right Side Reset"=FALSE, "Left Upper Limit"=1.0, "Right Upper Limit"=1.0, "Left Lower Limit"=-1.0, "Right Lower Limit"=-1.0) -> ("Encoder Status"=w690:T1, "Encoder Status 2"=w689:T1, "Encoder Status 3"=w688:T1)  [unwired: 8 in]
            n300 = Unbundle(w689) -> ()  [unwired: 4 out]
            n301 = Unbundle(w690) -> ("Encoder Distance"=w676:dbl)  [unwired: 3 out]
            "Left Distance 4" <- w676
            n302 = Unbundle(w688) -> ("Encoder Distance"=w674:dbl)  [unwired: 3 out]
            "Right Distance 4" <- w674
            n303 = Round To Nearest(number=w674) -> (nearest integer value=w686:dbl)
            n304 = Round To Nearest(number=w676) -> (nearest integer value=w683:dbl)
            n305 = Equal?(x=w686, y=18.0) -> (x = y?=w685:bool)
            n306 = Equal?(x=w683, y=0.0) -> (x = y?=w682:bool)
            n307 = And(x=w682, y=w685) -> (x .and. y?=w675:bool)
            n308 = call "Auto Arm Control.vi"("Upper Arm Rollers"=0.0, "Upper Arms Open"=FALSE, "Upper Arms Close"=FALSE, "Lower Roller Left"=w679, "Lower Roller Right"=w679, "Lower Arm Extend"=FALSE, "Lower Arm Retract"=FALSE) -> ()  [unwired: 9 in]
            "Stage 4" <- 4
          }
        }
        frame #4 {
          n309 = while {
            stop <- w712 stop-if-true
            w704 = 0.0
            w719 = -80.0
            # "Move forward 80\""
            n310 = call "Auto Drive Elev.vi"("Left Side Speed"=w719, "Right Side Speed"=w719, "Elevator Height"=32.0, "Left Side Reset"=FALSE, "Right Side Reset"=FALSE, "Left Upper Limit"=1.0, "Right Upper Limit"=1.0, "Left Lower Limit"=-1.0, "Right Lower Limit"=-1.0) -> ("Encoder Status"=w717:T1, "Encoder Status 2"=w716:T1, "Encoder Status 3"=w715:T1)  [unwired: 8 in]
            n311 = Unbundle(w716) -> ("Encoder Distance"=w701:dbl)  [unwired: 3 out]
            "Right Distance 5" <- w701
            n312 = Unbundle(w717) -> ("Encoder Distance"=w700:dbl)  [unwired: 3 out]
            "Left Distance 5" <- w700
            n313 = Unbundle(w715) -> ()  [unwired: 4 out]
            n314 = Round To Nearest(number=w701) -> (nearest integer value=w713:dbl)
            n315 = Round To Nearest(number=w700) -> (nearest integer value=w709:dbl)
            n316 = Equal?(x=w713, y=-80.0) -> (x = y?=w711:bool)
            n317 = Equal?(x=w709, y=-80.0) -> (x = y?=w708:bool)
            n318 = And(x=w708, y=w711) -> (x .and. y?=w712:bool)
            n319 = call "Auto Arm Control.vi"("Upper Arm Rollers"=0.0, "Upper Arms Open"=FALSE, "Upper Arms Close"=FALSE, "Lower Roller Left"=w704, "Lower Roller Right"=w704, "Lower Arm Extend"=FALSE, "Lower Arm Retract"=FALSE) -> ()  [unwired: 9 in]
            "Stage 5" <- 5
          }
        }
        frame #5 {
          n320 = while {
            stop <- w727 stop-if-true
            w732 = 0.0
            (unwired) FALSE
            w745 = -80.0
            # "Lower to  9\", release barrel"
            n321 = call "Auto Drive Elev.vi"("Left Side Speed"=w745, "Right Side Speed"=w745, "Elevator Height"=9.0, "Left Side Reset"=FALSE, "Right Side Reset"=FALSE, "Left Upper Limit"=1.0, "Right Upper Limit"=1.0, "Left Lower Limit"=-1.0, "Right Lower Limit"=-1.0) -> ("Encoder Status"=w743:T1, "Encoder Status 2"=w742:T1, "Encoder Status 3"=w741:T1)  [unwired: 8 in]
            n322 = Unbundle(w742) -> ()  [unwired: 4 out]
            n323 = Unbundle(w743) -> ("Encoder Distance"=w729:dbl)  [unwired: 3 out]
            "Left Distance 6" <- w729
            n324 = Unbundle(w741) -> ("Encoder Distance"=w728:dbl)  [unwired: 3 out]
            "Elev Height 6" <- w728
            n325 = Round To Nearest(number=w728) -> (nearest integer value=w739:dbl)
            n326 = Round To Nearest(number=w729) -> (nearest integer value=w736:dbl)
            n327 = Equal?(x=w739, y=9.0) -> (x = y?=w738:bool)
            n328 = Equal?(x=w736, y=-80.0) -> (x = y?=w735:bool)
            n329 = And(x=w735, y=w738) -> (x .and. y?=w727:bool)
            n330 = call "Auto Arm Control.vi"("Upper Arm Rollers"=0.0, "Upper Arms Open"=w727, "Upper Arms Close"=FALSE, "Lower Roller Left"=w732, "Lower Roller Right"=w732, "Lower Arm Extend"=FALSE, "Lower Arm Retract"=FALSE) -> ()  [unwired: 9 in]
            "Stage 6" <- 6
          }
        }
        frame #6 {
          n331 = Wait (ms)(milliseconds to wait=1) -> ()  [unwired: 1 out]
          "Stage 7" <- 7
        }
        frame #7 {
          n332 = while {
            stop <- w769 stop-if-true
            w756 = TRUE
            w761 = 0.0
            w776 = -72.0
            # "Shift upward"
            n333 = Not(x=w756) -> (.not. x?=w755:bool)
            n334 = call "Auto Drive Elev.vi"("Left Side Speed"=w776, "Right Side Speed"=w776, "Elevator Height"=9.0, "Left Side Reset"=FALSE, "Right Side Reset"=FALSE, "Left Upper Limit"=1.0, "Right Upper Limit"=1.0, "Left Lower Limit"=-1.0, "Right Lower Limit"=-1.0, "Up Shift"=w756, "Down Shift"=w755) -> ("Encoder Status"=w774:T1, "Encoder Status 2"=w773:T1, "Encoder Status 3"=w772:T1)  [unwired: 6 in]
            n335 = Unbundle(w773) -> ("Encoder Distance"=w758:dbl)  [unwired: 3 out]
            "Right Distance 8" <- w758
            n336 = Unbundle(w774) -> ("Encoder Distance"=w757:dbl)  [unwired: 3 out]
            "Left Distance 8" <- w757
            n337 = Unbundle(w772) -> ()  [unwired: 4 out]
            n338 = Round To Nearest(number=w758) -> (nearest integer value=w770:dbl)
            n339 = Round To Nearest(number=w757) -> (nearest integer value=w766:dbl)
            n340 = Equal?(x=w770, y=-72.0) -> (x = y?=w768:bool)
            n341 = Equal?(x=w766, y=-72.0) -> (x = y?=w765:bool)
            n342 = And(x=w765, y=w768) -> (x .and. y?=w769:bool)
            n343 = call "Auto Arm Control.vi"("Upper Arm Rollers"=0.0, "Upper Arms Open"=FALSE, "Upper Arms Close"=FALSE, "Lower Roller Left"=w761, "Lower Roller Right"=w761, "Lower Arm Extend"=FALSE, "Lower Arm Retract"=FALSE) -> ()  [unwired: 9 in]
            "Stage 8" <- 8
          }
        }
      }
    }
    frame 5 {
      # "1"
      n344 = flat-sequence {
        frame #0 {
          # "1"
          n345 = while {
            stop <- w785 stop-if-true
            w783 = FALSE
            w787 = 0.0
            (unwired) FALSE
            w803 = 0.0
            # "Reset"
            n346 = Not(x=w783) -> (.not. x?=w784:bool)
            n347 = call "Auto Drive Elev.vi"("Left Side Speed"=w803, "Right Side Speed"=w803, "Elevator Height"=9.0, "Left Side Reset"=TRUE, "Right Side Reset"=TRUE, "Left Upper Limit"=1.0, "Right Upper Limit"=1.0, "Left Lower Limit"=-1.0, "Right Lower Limit"=-1.0, "Up Shift"=w783, "Down Shift"=w784) -> ("Encoder Status"=w801:T1, "Encoder Status 2"=w800:T1, "Encoder Status 3"=w799:T1)  [unwired: 6 in]
            n348 = Unbundle(w800) -> ("Encoder Distance"=w796:dbl)  [unwired: 3 out]
            n349 = Unbundle(w801) -> ("Encoder Distance"=w792:dbl)  [unwired: 3 out]
            n350 = Unbundle(w799) -> ()  [unwired: 4 out]
            n351 = Round To Nearest(number=w796) -> (nearest integer value=w797:dbl)
            n352 = Round To Nearest(number=w792) -> (nearest integer value=w793:dbl)
            n353 = Equal?(x=w797, y=0.0) -> (x = y?=w795:bool)
            n354 = Equal?(x=w793, y=0.0) -> (x = y?=w791:bool)
            n355 = And(x=w791, y=w795) -> (x .and. y?=w785:bool)
            n356 = call "Auto Arm Control.vi"("Upper Arm Rollers"=0.0, "Upper Arms Open"=w785, "Upper Arms Close"=FALSE, "Lower Roller Left"=w787, "Lower Roller Right"=w787, "Lower Arm Extend"=FALSE, "Lower Arm Retract"=FALSE) -> ()  [unwired: 9 in]
          }
        }
        frame #1 {
          # "2"
          n357 = Wait (ms)(milliseconds to wait=1000) -> ()  [unwired: 1 out]
        }
        frame #2 {
          # "3"
          # "1"
          n358 = while {
            stop <- w812 stop-if-true
            w813 = 0.0
            (unwired) FALSE
            w829 = 0.0
            # "Raise upper arms at 9\" and close upper arms"
            n359 = call "Auto Drive Elev.vi"("Left Side Speed"=w829, "Right Side Speed"=w829, "Elevator Height"=9.0, "Left Side Reset"=TRUE, "Right Side Reset"=TRUE, "Left Upper Limit"=1.0, "Right Upper Limit"=1.0, "Left Lower Limit"=-1.0, "Right Lower Limit"=-1.0) -> ("Encoder Status"=w827:T1, "Encoder Status 2"=w826:T1, "Encoder Status 3"=w825:T1)  [unwired: 8 in]
            n360 = Unbundle(w826) -> ()  [unwired: 4 out]
            n361 = Unbundle(w827) -> ("Encoder Distance"=w819:dbl)  [unwired: 3 out]
            n362 = Unbundle(w825) -> ("Encoder Distance"=w816:dbl)  [unwired: 3 out]
            n363 = Round To Nearest(number=w816) -> (nearest integer value=w823:dbl)
            n364 = Round To Nearest(number=w819) -> (nearest integer value=w820:dbl)
            n365 = Equal?(x=w823, y=9.0) -> (x = y?=w822:bool)
            n366 = Equal?(x=w820, y=0.0) -> (x = y?=w811:bool)
            n367 = And(x=w811, y=w822) -> (x .and. y?=w812:bool)
            n368 = call "Auto Arm Control.vi"("Upper Arm Rollers"=0.0, "Upper Arms Open"=FALSE, "Upper Arms Close"=w812, "Lower Roller Left"=w813, "Lower Roller Right"=w813, "Lower Arm Extend"=FALSE, "Lower Arm Retract"=FALSE) -> ()  [unwired: 9 in]
          }
        }
        frame #3 {
          # "4"
          n369 = Wait (ms)(milliseconds to wait=1000) -> ()  [unwired: 1 out]
        }
        frame #4 {
          # "5"
          n370 = while {
            stop <- w849 stop-if-true
            w838 = 0.0
            w856 = 0.0
            # "Raise Upper Arms to 32\""
            n371 = call "Auto Drive Elev.vi"("Left Side Speed"=w856, "Right Side Speed"=w856, "Elevator Height"=32.0, "Left Side Reset"=FALSE, "Right Side Reset"=FALSE, "Left Upper Limit"=1.0, "Right Upper Limit"=1.0, "Left Lower Limit"=-1.0, "Right Lower Limit"=-1.0) -> ("Encoder Status"=w854:T1, "Encoder Status 2"=w853:T1, "Encoder Status 3"=w852:T1)  [unwired: 8 in]
            n372 = Unbundle(w853) -> ()  [unwired: 4 out]
            n373 = Unbundle(w854) -> ("Encoder Distance"=w845:dbl)  [unwired: 3 out]
            n374 = Unbundle(w852) -> ("Encoder Distance"=w840:dbl)  [unwired: 3 out]
            n375 = Round To Nearest(number=w840) -> (nearest integer value=w850:dbl)
            n376 = Round To Nearest(number=w845) -> (nearest integer value=w846:dbl)
            n377 = Equal?(x=w850, y=32.0) -> (x = y?=w848:bool)
            n378 = Equal?(x=w846, y=0.0) -> (x = y?=w844:bool)
            n379 = And(x=w844, y=w848) -> (x .and. y?=w849:bool)
            n380 = call "Auto Arm Control.vi"("Upper Arm Rollers"=0.0, "Upper Arms Open"=FALSE, "Upper Arms Close"=FALSE, "Lower Roller Left"=w838, "Lower Roller Right"=w838, "Lower Arm Extend"=FALSE, "Lower Arm Retract"=FALSE) -> ()  [unwired: 9 in]
          }
        }
        frame #5 {
          # "6"
          n381 = while {
            stop <- w874 stop-if-true
            w863 = 0.0
            w882 = 24.0
            # "Move forward 24\""
            n382 = call "Auto Drive Elev.vi"("Left Side Speed"=w882, "Right Side Speed"=w882, "Elevator Height"=32.0, "Left Side Reset"=FALSE, "Right Side Reset"=FALSE, "Left Upper Limit"=1.0, "Right Upper Limit"=1.0, "Left Lower Limit"=-1.0, "Right Lower Limit"=-1.0) -> ("Encoder Status"=w880:T1, "Encoder Status 2"=w879:T1, "Encoder Status 3"=w878:T1)  [unwired: 8 in]
            n383 = Unbundle(w879) -> ("Encoder Distance"=w875:dbl)  [unwired: 3 out]
            n384 = Unbundle(w880) -> ("Encoder Distance"=w870:dbl)  [unwired: 3 out]
            n385 = Unbundle(w878) -> ()  [unwired: 4 out]
            n386 = Round To Nearest(number=w875) -> (nearest integer value=w876:dbl)
            n387 = Round To Nearest(number=w870) -> (nearest integer value=w871:dbl)
            n388 = Equal?(x=w876, y=24.0) -> (x = y?=w873:bool)
            n389 = Equal?(x=w871, y=24.0) -> (x = y?=w869:bool)
            n390 = And(x=w869, y=w873) -> (x .and. y?=w874:bool)
            n391 = call "Auto Arm Control.vi"("Upper Arm Rollers"=0.0, "Upper Arms Open"=FALSE, "Upper Arms Close"=FALSE, "Lower Roller Left"=w863, "Lower Roller Right"=w863, "Lower Arm Extend"=FALSE, "Lower Arm Retract"=FALSE) -> ()  [unwired: 9 in]
          }
        }
        frame #6 {
          # "7"
          n392 = while {
            stop <- w889 stop-if-true
            w890 = 0.0
            (unwired) FALSE
            w907 = 24.0
            # "Lower barrel to 30\", release barrel"
            n393 = call "Auto Drive Elev.vi"("Left Side Speed"=w907, "Right Side Speed"=w907, "Elevator Height"=30.0, "Left Side Reset"=FALSE, "Right Side Reset"=FALSE, "Left Upper Limit"=1.0, "Right Upper Limit"=1.0, "Left Lower Limit"=-1.0, "Right Lower Limit"=-1.0) -> ("Encoder Status"=w905:T1, "Encoder Status 2"=w904:T1, "Encoder Status 3"=w903:T1)  [unwired: 8 in]
            n394 = Unbundle(w904) -> ()  [unwired: 4 out]
            n395 = Unbundle(w905) -> ("Encoder Distance"=w897:dbl)  [unwired: 3 out]
            n396 = Unbundle(w903) -> ("Encoder Distance"=w893:dbl)  [unwired: 3 out]
            n397 = Round To Nearest(number=w893) -> (nearest integer value=w901:dbl)
            n398 = Round To Nearest(number=w897) -> (nearest integer value=w898:dbl)
            n399 = Equal?(x=w901, y=30.0) -> (x = y?=w900:bool)
            n400 = Equal?(x=w898, y=24.0) -> (x = y?=w896:bool)
            n401 = And(x=w896, y=w900) -> (x .and. y?=w889:bool)
            n402 = call "Auto Arm Control.vi"("Upper Arm Rollers"=0.0, "Upper Arms Open"=w889, "Upper Arms Close"=FALSE, "Lower Roller Left"=w890, "Lower Roller Right"=w890, "Lower Arm Extend"=FALSE, "Lower Arm Retract"=FALSE) -> ()  [unwired: 9 in]
          }
        }
        frame #7 {
          # "8"
          n403 = Wait (ms)(milliseconds to wait=1000) -> ()  [unwired: 1 out]
        }
        frame #8 {
          # "8"
          n404 = while {
            stop <- w915 stop-if-true
            w918 = 0.0
            (unwired) FALSE
            w933 = 24.0
            # "Lower upper arms to 9\", grab tote"
            n405 = call "Auto Drive Elev.vi"("Left Side Speed"=w933, "Right Side Speed"=w933, "Elevator Height"=9.0, "Left Side Reset"=FALSE, "Right Side Reset"=FALSE, "Left Upper Limit"=1.0, "Right Upper Limit"=1.0, "Left Lower Limit"=-1.0, "Right Lower Limit"=-1.0) -> ("Encoder Status"=w931:T1, "Encoder Status 2"=w930:T1, "Encoder Status 3"=w929:T1)  [unwired: 8 in]
            n406 = Unbundle(w930) -> ()  [unwired: 4 out]
            n407 = Unbundle(w931) -> ("Encoder Distance"=w923:dbl)  [unwired: 3 out]
            n408 = Unbundle(w929) -> ("Encoder Distance"=w919:dbl)  [unwired: 3 out]
            n409 = Round To Nearest(number=w919) -> (nearest integer value=w927:dbl)
            n410 = Round To Nearest(number=w923) -> (nearest integer value=w924:dbl)
            n411 = Equal?(x=w927, y=9.0) -> (x = y?=w926:bool)
            n412 = Equal?(x=w924, y=24.0) -> (x = y?=w922:bool)
            n413 = And(x=w922, y=w926) -> (x .and. y?=w915:bool)
            n414 = call "Auto Arm Control.vi"("Upper Arm Rollers"=0.0, "Upper Arms Open"=FALSE, "Upper Arms Close"=w915, "Lower Roller Left"=w918, "Lower Roller Right"=w918, "Lower Arm Extend"=FALSE, "Lower Arm Retract"=FALSE) -> ()  [unwired: 9 in]
          }
        }
        frame #9 {
          # "9"
          n415 = Wait (ms)(milliseconds to wait=1000) -> ()  [unwired: 1 out]
        }
        frame #10 {
          # "10"
          n416 = while {
            stop <- w953 stop-if-true
            w941 = 0.0
            w960 = 24.0
            # "Raise tote/barrel to 18\""
            n417 = call "Auto Drive Elev.vi"("Left Side Speed"=w960, "Right Side Speed"=w960, "Elevator Height"=18.0, "Left Side Reset"=TRUE, "Right Side Reset"=TRUE, "Left Upper Limit"=1.0, "Right Upper Limit"=1.0, "Left Lower Limit"=-1.0, "Right Lower Limit"=-1.0) -> ("Encoder Status"=w958:T1, "Encoder Status 2"=w957:T1, "Encoder Status 3"=w956:T1)  [unwired: 8 in]
            n418 = Unbundle(w957) -> ()  [unwired: 4 out]
            n419 = Unbundle(w958) -> ("Encoder Distance"=w949:dbl)  [unwired: 3 out]
            n420 = Unbundle(w956) -> ("Encoder Distance"=w944:dbl)  [unwired: 3 out]
            n421 = Round To Nearest(number=w944) -> (nearest integer value=w954:dbl)
            n422 = Round To Nearest(number=w949) -> (nearest integer value=w950:dbl)
            n423 = Equal?(x=w954, y=18.0) -> (x = y?=w952:bool)
            n424 = Equal?(x=w950, y=0.0) -> (x = y?=w945:bool)
            n425 = And(x=w945, y=w952) -> (x .and. y?=w953:bool)
            n426 = call "Auto Arm Control.vi"("Upper Arm Rollers"=0.0, "Upper Arms Open"=FALSE, "Upper Arms Close"=FALSE, "Lower Roller Left"=w941, "Lower Roller Right"=w941, "Lower Arm Extend"=FALSE, "Lower Arm Retract"=FALSE) -> ()  [unwired: 9 in]
          }
        }
        frame #11 {
          # "11"
          n427 = while {
            stop <- w981 stop-if-true
            w967 = 0.0
            w970 = 28.0
            # "Turn left 90 degrees"
            n428 = Negate(x=w970) -> (-x=w971:dbl)
            n429 = call "Auto Drive Elev.vi"("Left Side Speed"=w971, "Right Side Speed"=w970, "Elevator Height"=18.0, "Left Side Reset"=FALSE, "Right Side Reset"=FALSE, "Left Upper Limit"=1.0, "Right Upper Limit"=1.0, "Left Lower Limit"=-1.0, "Right Lower Limit"=-1.0) -> ("Encoder Status"=w986:T1, "Encoder Status 2"=w985:T1, "Encoder Status 3"=w984:T1)  [unwired: 8 in]
            n430 = Unbundle(w985) -> ("Encoder Distance"=w972:dbl)  [unwired: 3 out]
            n431 = Unbundle(w986) -> ("Encoder Distance"=w977:dbl)  [unwired: 3 out]
            n432 = Unbundle(w984) -> ()  [unwired: 4 out]
            n433 = Round To Nearest(number=w972) -> (nearest integer value=w982:dbl)
            n434 = Round To Nearest(number=w977) -> (nearest integer value=w978:dbl)
            n435 = Equal?(x=w982, y=28.0) -> (x = y?=w980:bool)
            n436 = Equal?(x=w978, y=-28.0) -> (x = y?=w973:bool)
            n437 = And(x=w973, y=w980) -> (x .and. y?=w981:bool)
            n438 = call "Auto Arm Control.vi"("Upper Arm Rollers"=0.0, "Upper Arms Open"=FALSE, "Upper Arms Close"=FALSE, "Lower Roller Left"=w967, "Lower Roller Right"=w967, "Lower Arm Extend"=FALSE, "Lower Arm Retract"=FALSE) -> ()  [unwired: 9 in]
          }
        }
        frame #12 {
          # "12"
          n439 = while {
            stop <- w1007 stop-if-true
            w996 = 28.0
            # "Reset drivetrain"
            n440 = Negate(x=w996) -> (-x=w997:dbl)
            n441 = call "Auto Drive Elev.vi"("Left Side Speed"=w997, "Right Side Speed"=w996, "Elevator Height"=18.0, "Left Side Reset"=TRUE, "Right Side Reset"=TRUE, "Left Upper Limit"=1.0, "Right Upper Limit"=1.0, "Left Lower Limit"=-1.0, "Right Lower Limit"=-1.0) -> ("Encoder Status"=w1012:T1, "Encoder Status 2"=w1011:T1, "Encoder Status 3"=w1010:T1)  [unwired: 8 in]
            n442 = Unbundle(w1011) -> ("Encoder Distance"=w998:dbl)  [unwired: 3 out]
            n443 = Unbundle(w1012) -> ("Encoder Distance"=w1003:dbl)  [unwired: 3 out]
            n444 = Unbundle(w1010) -> ()  [unwired: 4 out]
            n445 = Round To Nearest(number=w998) -> (nearest integer value=w1008:dbl)
            n446 = Round To Nearest(number=w1003) -> (nearest integer value=w1004:dbl)
            n447 = Equal?(x=w1008, y=0.0) -> (x = y?=w1006:bool)
            n448 = Equal?(x=w1004, y=0.0) -> (x = y?=w999:bool)
            n449 = And(x=w999, y=w1006) -> (x .and. y?=w1007:bool)
            n450 = call "Auto Arm Control.vi"("Upper Arm Rollers"=0.0, "Upper Arms Open"=FALSE, "Upper Arms Close"=FALSE, "Lower Arm Extend"=FALSE, "Lower Arm Retract"=FALSE) -> ()  [unwired: 11 in]
          }
        }
        frame #13 {
          # "13"
          n451 = while {
            stop <- w1032 stop-if-true
            w1022 = 80.0
            # "Move forward 80\""
            n452 = call "Auto Drive Elev.vi"("Left Side Speed"=w1022, "Right Side Speed"=w1022, "Elevator Height"=18.0, "Left Side Reset"=FALSE, "Right Side Reset"=FALSE, "Left Upper Limit"=1.0, "Right Upper Limit"=1.0, "Left Lower Limit"=-1.0, "Right Lower Limit"=-1.0) -> ("Encoder Status"=w1037:T1, "Encoder Status 2"=w1036:T1, "Encoder Status 3"=w1035:T1)  [unwired: 8 in]
            n453 = Unbundle(w1036) -> ("Encoder Distance"=w1023:dbl)  [unwired: 3 out]
            n454 = Unbundle(w1037) -> ("Encoder Distance"=w1028:dbl)  [unwired: 3 out]
            n455 = Unbundle(w1035) -> ()  [unwired: 4 out]
            n456 = Round To Nearest(number=w1023) -> (nearest integer value=w1033:dbl)
            n457 = Round To Nearest(number=w1028) -> (nearest integer value=w1029:dbl)
            n458 = Equal?(x=w1033, y=80.0) -> (x = y?=w1031:bool)
            n459 = Equal?(x=w1029, y=80.0) -> (x = y?=w1024:bool)
            n460 = And(x=w1024, y=w1031) -> (x .and. y?=w1032:bool)
            n461 = call "Auto Arm Control.vi"("Upper Arm Rollers"=0.0, "Upper Arms Open"=FALSE, "Upper Arms Close"=FALSE, "Lower Arm Extend"=FALSE, "Lower Arm Retract"=FALSE) -> ()  [unwired: 11 in]
          }
        }
        frame #14 {
          # "14"
          n462 = while {
            stop <- w1045 stop-if-true
            (unwired) FALSE
            w1049 = 80.0
            # "Lower tote/barrel to 9\", release tote/barrel"
            n463 = call "Auto Drive Elev.vi"("Left Side Speed"=w1049, "Right Side Speed"=w1049, "Elevator Height"=9.0, "Left Side Reset"=FALSE, "Right Side Reset"=FALSE, "Left Upper Limit"=1.0, "Right Upper Limit"=1.0, "Left Lower Limit"=-1.0, "Right Lower Limit"=-1.0) -> ("Encoder Status"=w1061:T1, "Encoder Status 2"=w1060:T1, "Encoder Status 3"=w1059:T1)  [unwired: 8 in]
            n464 = Unbundle(w1060) -> ()  [unwired: 4 out]
            n465 = Unbundle(w1061) -> ("Encoder Distance"=w1053:dbl)  [unwired: 3 out]
            n466 = Unbundle(w1059) -> ("Encoder Distance"=w1048:dbl)  [unwired: 3 out]
            n467 = Round To Nearest(number=w1048) -> (nearest integer value=w1057:dbl)
            n468 = Round To Nearest(number=w1053) -> (nearest integer value=w1054:dbl)
            n469 = Equal?(x=w1057, y=9.0) -> (x = y?=w1056:bool)
            n470 = Equal?(x=w1054, y=80.0) -> (x = y?=w1050:bool)
            n471 = And(x=w1050, y=w1056) -> (x .and. y?=w1045:bool)
            n472 = call "Auto Arm Control.vi"("Upper Arm Rollers"=0.0, "Upper Arms Open"=w1045, "Upper Arms Close"=FALSE, "Lower Arm Extend"=FALSE, "Lower Arm Retract"=FALSE) -> ()  [unwired: 11 in]
          }
        }
        frame #15 {
          # "14"
          n473 = Wait (ms)(milliseconds to wait=1000) -> ()  [unwired: 1 out]
        }
        frame #16 {
          # "14"
          n474 = while {
            stop <- w1085 stop-if-true
            w1070 = TRUE
            w1072 = 0.0
            w1075 = FALSE
            w1078 = 80.0
            # "Finish"
            n475 = Not(x=w1070) -> (.not. x?=w1071:bool)
            n476 = call "Auto Drive Elev.vi"("Left Side Speed"=w1078, "Right Side Speed"=w1078, "Elevator Height"=9.0, "Left Side Reset"=FALSE, "Right Side Reset"=FALSE, "Left Upper Limit"=1.0, "Right Upper Limit"=1.0, "Left Lower Limit"=-1.0, "Right Lower Limit"=-1.0, "Up Shift"=w1070, "Down Shift"=w1071) -> ("Encoder Status"=w1090:T1, "Encoder Status 2"=w1089:T1, "Encoder Status 3"=w1088:T1)  [unwired: 6 in]
            n477 = Unbundle(w1089) -> ()  [unwired: 4 out]
            n478 = Unbundle(w1090) -> ("Encoder Distance"=w1081:dbl)  [unwired: 3 out]
            n479 = Unbundle(w1088) -> ("Encoder Distance"=w1077:dbl)  [unwired: 3 out]
            n480 = Round To Nearest(number=w1077) -> (nearest integer value=w1086:dbl)
            n481 = Round To Nearest(number=w1081) -> (nearest integer value=w1082:dbl)
            n482 = Equal?(x=w1086, y=9.0) -> (x = y?=w1084:bool)
            n483 = Equal?(x=w1082, y=80.0) -> ()  [unwired: 1 out]
            n484 = Not(x=w1075) -> (.not. x?=w1076:bool)
            n485 = And(x=w1076, y=w1084) -> (x .and. y?=w1085:bool)
            n486 = call "Auto Arm Control.vi"("Upper Arm Rollers"=0.0, "Upper Arms Open"=w1075, "Upper Arms Close"=FALSE, "Lower Roller Left"=w1072, "Lower Roller Right"=w1072, "Lower Arm Extend"=FALSE, "Lower Arm Retract"=FALSE) -> ()  [unwired: 9 in]
          }
        }
      }
    }
  }
  n487 = call <vilib>:"WPI_DriverStationGet Alliance Info.vi"() -> ()  [unwired: 12 out]
  n488 = call <vilib>:"WPI_JoystickRefNum Registry Get.vi"("refnum name"="Joystick 0") -> ("JoystickDevRef"=w4:T2)  [unwired: 1 in, 9 out]
  n489 = call <vilib>:"WPI_JoystickGetValues.vi"("JoystickDevRef"=w4) -> ("Axes"=w2:dbl[])  [unwired: 6 in, 4 out]
  n490 = call <vilib>:"SD Write Numeric Array.vi"("Numeric Array"=w2, "Name"="Joystick 0/Axes") -> ()  [unwired: 8 in, 2 out]
  n491 = while {
    stop <- FALSE stop-if-true
    n492 = call <vilib>:"WPI_DriverStationReport Robot Code State.vi"("Autonomous"=TRUE) -> ()  [unwired: 10 in, 1 out]
    n493 = Wait (ms)(milliseconds to wait=u32 20) -> ()  [unwired: 1 out]
  }
